vi "Compare Request and Response.vi"(8 "error in (no error)":errorcluster, 9 "JSON Response String":string, 10 "JSON Request String":string, 11 "ServerTest in":refnum<class "ServerTest.lvclass">) -> (0 "error out":errorcluster, 3 "ServerTest out":refnum<class "ServerTest.lvclass">)   [LabVIEW 2017, in "ServerTest.lvclass"]
uses:
  ServerTest.lvclass
  C:/Program Files (x86)/National Instruments/LabVIEW 2017/vi.lib/addons/_JKI Toolkits/VI Tester/TestCase.llb/TestCase.lvclass
  Classes/Server/Send Request (Sync).vi
  Classes/Server/JSONRPC Server.lvclass
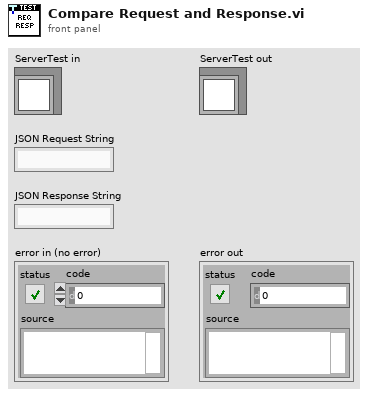
[diagram p1: front panel]
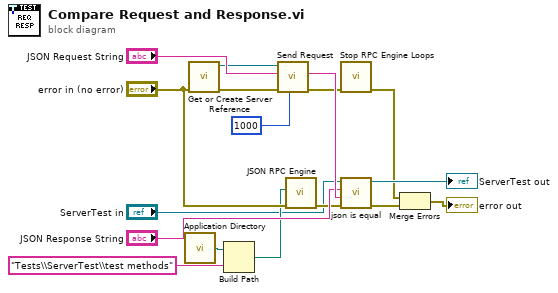
[diagram p0: block diagram]
diagram:
  n1 = call <vilib>:"Application Directory.vi"() -> ("Application Directory"=w5:path)
  n2 = call "Get or Create Server Reference.vi"("error in (no error)"="error in (no error)") -> ("error out"=w17:errorcluster, "Server Out"=w8:refnum<class "JSONRPC Server.lvclass">)  [unwired: 9 in]
  n3 = Build Path(base path=w5, name or relative path="Tests\\ServerTest\\test methods") -> (appended path=w7:path)
  n4 = call-poly "Send Request.vi"("Timeout in ms(-1)"=1000, "error in (no error)"=w17, "JSON Request String"="JSON Request String", "JSONRPC Server in"=w8) -> ("error out"=w12:errorcluster, "JSON Response String"=w15:string)  [unwired: 5 in, 1 out]
  n5 = call "JSON RPC Engine.vi"("error in (no error)"="error in (no error)", "methods directory"=w7) -> ("error out"=w11:errorcluster)  [unwired: 9 in]
  n6 = call "Stop RPC Engine Loops.vi"("error in (no error)"=w12) -> ("error out"=w1:errorcluster)  [unwired: 10 in]
  n7 = call "json is equal.vi"("error in (no error)"=w11, "json string B"=w15, "json string A"="JSON Response String", "TestCase in"="ServerTest in") -> ("error out"=w13:errorcluster, "TestCase out"=→"ServerTest out":refnum<class "ServerTest.lvclass">)  [unwired: 6 in]
  n8 = Merge Errors(w1, w13) -> (→"error out":errorcluster)
